vi "HW_Timings_Calibration.vi"(3 "Error In":errorcluster, 4 "Calibration SW timings":dbl[](array[numeric]), 5 "Calibration HW timings":u32[](array[numeric]), 6 "Settings cluster in":T1={"Defaults"={"Default User"=0.0, "VISA Resource Name "="Tracker"}, "Recording and saving"={"Researcher name"="Researcher", "Name prefix"="Track", "Data post-processing"={"Filter type"=enum."Savitzky-Golay", "Length"=31, "Order"=3}, "Stop at"=0.0, "\"Stop at\" enabled"=FALSE, "Default save folder path"=path "", "Acquisition FPS"=enum."Optimal"}, "Geometry"={"Cage diameter, mm"=180, "Starting angle MIDFIELD"=0, "Starting angle BORDER"=0, "Radius, mm CENTER"=30, "Radius, mm MIDFIELD"=75, "N segments MIDFIELD"=2, "N segments BORDER"=4, "R-gap, mm"=0.0, "Bridge swap"=FALSE, "Bridge H. offset"=0.0, "Bridge V. offset"=0.0, "Twisted neck"=FALSE, "Alt. magn. orientation"=FALSE}, "IO parameters"={"IO general config."=12, "IO 1 configuration"=1, "IO 2 configuration"=1, "IO 3 configuration"=0, "IO 4 configuration"=0, "Activate ext. RS-232"=0, "IO inversion config."=0, "Sync capability"=1}, "Stimulus presets array"=[{"Event type"=0, "Dur., s"=0.0, "Stim., s"=0.0, "TTL out N"=1, "Set/Clear"=FALSE, "Stim. has been set"=FALSE}, {"Event type"=0, "Dur., s"=0.0, "Stim., s"=0.0, "TTL out N"=1, "Set/Clear"=FALSE, "Stim. has been set"=FALSE}, {"Event type"=0, "Dur., s"=0.0, "Stim., s"=0.0, "TTL out N"=1, "Set/Clear"=FALSE, "Stim. has been set"=FALSE}, {"Event type"=0, "Dur., s"=0.0, "Stim., s"=0.0, "TTL out N"=1, "Set/Clear"=FALSE, "Stim. has been set"=FALSE}, {"Event type"=0, "Dur., s"=0.0, "Stim., s"=0.0, "TTL out N"=1, "Set/Clear"=FALSE, "Stim. has been set"=FALSE}, {"Event type"=0, "Dur., s"=0.0, "Stim., s"=0.0, "TTL out N"=1, "Set/Clear"=FALSE, "Stim. has been set"=FALSE}, {"Event type"=0, "Dur., s"=0.0, "Stim., s"=0.0, "TTL out N"=1, "Set/Clear"=FALSE, "Stim. has been set"=FALSE}, {"Event type"=0, "Dur., s"=0.0, "Stim., s"=0.0, "TTL out N"=1, "Set/Clear"=FALSE, "Stim. has been set"=FALSE}, {"Event type"=0, "Dur., s"=0.0, "Stim., s"=0.0, "TTL out N"=1, "Set/Clear"=FALSE, "Stim. has been set"=FALSE}, {"Event type"=0, "Dur., s"=0.0, "Stim., s"=0.0, "TTL out N"=1, "Set/Clear"=FALSE, "Stim. has been set"=FALSE}, {"Event type"=0, "Dur., s"=0.0, "Stim., s"=0.0, "TTL out N"=1, "Set/Clear"=FALSE, "Stim. has been set"=FALSE}, {"Event type"=0, "Dur., s"=0.0, "Stim., s"=0.0, "TTL out N"=1, "Set/Clear"=FALSE, "Stim. has been set"=FALSE}, {"Event type"=0, "Dur., s"=0.0, "Stim., s"=0.0, "TTL out N"=1, "Set/Clear"=FALSE, "Stim. has been set"=FALSE}, {"Event type"=0, "Dur., s"=0.0, "Stim., s"=0.0, "TTL out N"=1, "Set/Clear"=FALSE, "Stim. has been set"=FALSE}], "Calibration parameters"={"Timing calibration sw/hw"=1.0, "True FPS"=80.0, "Disp. calibration info"=[]}, "Settings loaded OK"=FALSE} {"Calibration parameters"."Disp. calibration info"."Speed, µl per ms" format="%.3g"; "Calibration parameters"."True FPS" format="%.10g"; "Calibration parameters"."Timing calibration sw/hw" format="%.10g"; "Stimulus presets array"."Event type" items=["Stay for N seconds"]; "Stimulus presets array"."TTL out N" items=["1"=1, "2"=2, "1+2"=3]; "Recording and saving"."Data post-processing"."Order" min=3 max=11 step=2; "Recording and saving"."Data post-processing"."Length" min=5 max=301 step=2; "Geometry"."Cage diameter, mm" scale=0.0..340.0}) -> (0 "Error out":T9, 1 "Calibration information":string, 2 "Settings cluster out":T1={"Defaults"={"Default User"=0.0, "VISA Resource Name "="Tracker"}, "Recording and saving"={"Researcher name"="Researcher", "Name prefix"="Track", "Data post-processing"={"Filter type"=enum."Savitzky-Golay", "Length"=31, "Order"=3}, "Stop at"=0.0, "\"Stop at\" enabled"=FALSE, "Default save folder path"=path "", "Acquisition FPS"=enum."Optimal"}, "Geometry"={"Cage diameter, mm"=180, "Starting angle MIDFIELD"=0, "Starting angle BORDER"=0, "Radius, mm CENTER"=30, "Radius, mm MIDFIELD"=75, "N segments MIDFIELD"=2, "N segments BORDER"=4, "R-gap, mm"=0.0, "Bridge swap"=FALSE, "Bridge H. offset"=0.0, "Bridge V. offset"=0.0, "Twisted neck"=FALSE, "Alt. magn. orientation"=FALSE}, "IO parameters"={"IO general config."=12, "IO 1 configuration"=1, "IO 2 configuration"=1, "IO 3 configuration"=0, "IO 4 configuration"=0, "Activate ext. RS-232"=0, "IO inversion config."=0, "Sync capability"=1}, "Stimulus presets array"=[{"Event type"=0, "Dur., s"=0.0, "Stim., s"=0.0, "TTL out N"=1, "Set/Clear"=FALSE, "Stim. has been set"=FALSE}, {"Event type"=0, "Dur., s"=0.0, "Stim., s"=0.0, "TTL out N"=1, "Set/Clear"=FALSE, "Stim. has been set"=FALSE}, {"Event type"=0, "Dur., s"=0.0, "Stim., s"=0.0, "TTL out N"=1, "Set/Clear"=FALSE, "Stim. has been set"=FALSE}, {"Event type"=0, "Dur., s"=0.0, "Stim., s"=0.0, "TTL out N"=1, "Set/Clear"=FALSE, "Stim. has been set"=FALSE}, {"Event type"=0, "Dur., s"=0.0, "Stim., s"=0.0, "TTL out N"=1, "Set/Clear"=FALSE, "Stim. has been set"=FALSE}, {"Event type"=0, "Dur., s"=0.0, "Stim., s"=0.0, "TTL out N"=1, "Set/Clear"=FALSE, "Stim. has been set"=FALSE}, {"Event type"=0, "Dur., s"=0.0, "Stim., s"=0.0, "TTL out N"=1, "Set/Clear"=FALSE, "Stim. has been set"=FALSE}, {"Event type"=0, "Dur., s"=0.0, "Stim., s"=0.0, "TTL out N"=1, "Set/Clear"=FALSE, "Stim. has been set"=FALSE}, {"Event type"=0, "Dur., s"=0.0, "Stim., s"=0.0, "TTL out N"=1, "Set/Clear"=FALSE, "Stim. has been set"=FALSE}, {"Event type"=0, "Dur., s"=0.0, "Stim., s"=0.0, "TTL out N"=1, "Set/Clear"=FALSE, "Stim. has been set"=FALSE}, {"Event type"=0, "Dur., s"=0.0, "Stim., s"=0.0, "TTL out N"=1, "Set/Clear"=FALSE, "Stim. has been set"=FALSE}, {"Event type"=0, "Dur., s"=0.0, "Stim., s"=0.0, "TTL out N"=1, "Set/Clear"=FALSE, "Stim. has been set"=FALSE}, {"Event type"=0, "Dur., s"=0.0, "Stim., s"=0.0, "TTL out N"=1, "Set/Clear"=FALSE, "Stim. has been set"=FALSE}, {"Event type"=0, "Dur., s"=0.0, "Stim., s"=0.0, "TTL out N"=1, "Set/Clear"=FALSE, "Stim. has been set"=FALSE}], "Calibration parameters"={"Timing calibration sw/hw"=1.0, "True FPS"=80.0, "Disp. calibration info"=[]}, "Settings loaded OK"=FALSE} {"Calibration parameters"."Disp. calibration info"."Speed, µl per ms" format="%.3g"; "Calibration parameters"."True FPS" format="%.10g"; "Calibration parameters"."Timing calibration sw/hw" format="%.10g"; "Stimulus presets array"."Event type" items=["Stay for N seconds"]; "Stimulus presets array"."TTL out N" items=["1"=1, "2"=2, "1+2"=3]; "Recording and saving"."Data post-processing"."Order" min=3 max=11 step=2; "Recording and saving"."Data post-processing"."Length" min=5 max=301 step=2; "Geometry"."Cage diameter, mm" scale=0.0..340.0})   [LabVIEW 2018, in "Tracker.lvlib"]
uses:
  Tracker.lvlib
  Controls/CTL_Settings_cluster.ctl
  Controls/CTL_Filter_selector.ctl
  Controls/CTL_Acquisition_speed_selector.ctl
  Controls/CTL_Segmented_plot_parameters.ctl
  Controls/CTL_IO_params_cluster.ctl
  Controls/CTL_Single_stimulus_setting.ctl
  Controls/CTL_Calibration_parameters.ctl
  Controls/CTL_Dispenser_calibration_info.ctl
  <vilib>/Utility/miscctls.llb/LVPointTypeDef.ctl
  <vilib>/Analysis/NI_AALBase.lvlib
panel:
  out "SW seconds in HW second":dbl format="%#.10g"
  in  "OK Button":bool
  out "True FPS":dbl format="%.3f"
  out "Avg. software frame time SD, ms":dbl format="%.3f"
  out "Avg. hardware frame time SD, ms":dbl format="%.3f"
  out "Avg. software frame time, ms":dbl format="%.3f"
  out "Avg. hardware frame time, ms":dbl format="%.3f"
  out "Frame delta time, ms":dbl[][](graph) caption="Waveform Chart - Light"
  # "Calibration information"
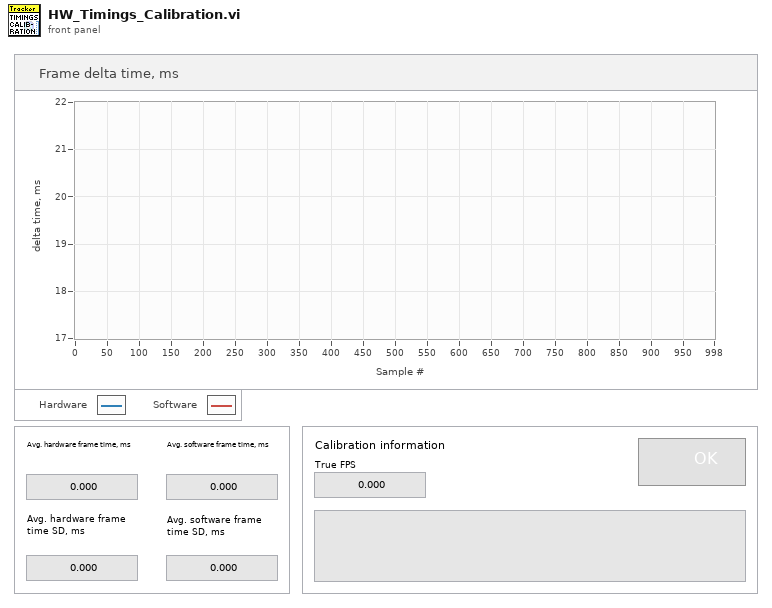
[diagram p1: front panel]
types:
  T1 = typedef "Tracker.lvlib/CTL_Settings_cluster.ctl" = cluster{"Defaults":cluster{"Default User":dbl, "VISA Resource Name ":string}, "Recording and saving":cluster{"Researcher name":string, "Name prefix":string, "Data post-processing":T2, "Stop at":dbl, "\"Stop at\" enabled":bool, "Default save folder path":path, "Acquisition FPS":T3}, "Geometry":T4, "IO parameters":T5, "Stimulus presets array":T6[], "Calibration parameters":T7, "Settings loaded OK":bool}
  T2 = typedef "Tracker.lvlib/CTL_Filter_selector.ctl" = cluster{"Filter type":enum16{"None", "Savitzky-Golay"}, "Length":i32, "Order":i32}
  T3 = typedef "Tracker.lvlib/CTL_Acquisition_speed_selector.ctl" = enum16{"Max", "Optimal", "Eco"}
  T4 = typedef "Tracker.lvlib/CTL_Segmented_plot_parameters.ctl" = cluster{"Cage diameter, mm":u16, "Starting angle MIDFIELD":i16, "Starting angle BORDER":i16, "Radius, mm CENTER":u16, "Radius, mm MIDFIELD":u16, "N segments MIDFIELD":u8, "N segments BORDER":u8, "R-gap, mm":sgl, "Bridge swap":bool, "Bridge H. offset":sgl, "Bridge V. offset":sgl, "Twisted neck":bool, "Alt. magn. orientation":bool}
  T5 = typedef "Tracker.lvlib/CTL_IO_params_cluster.ctl" = cluster{"IO general config.":u16, "IO 1 configuration":u16, "IO 2 configuration":u16, "IO 3 configuration":u16, "IO 4 configuration":u16, "Activate ext. RS-232":u16, "IO inversion config.":u16, "Sync capability":u8}
  T6 = typedef "Tracker.lvlib/CTL_Single_stimulus_setting.ctl" = cluster{"Event type":u16, "Dur., s":sgl, "Stim., s":sgl, "TTL out N":u16, "Set/Clear":bool, "Stim. has been set":bool}
  T7 = typedef "Tracker.lvlib/CTL_Calibration_parameters.ctl" = cluster{"Timing calibration sw/hw":dbl, "True FPS":dbl, "Disp. calibration info":T8}
  T8 = typedef "Tracker.lvlib/CTL_Dispenser_calibration_info.ctl" = cluster{"Channel":u8, "Speed, µl per ms":dbl}[]
  T9 = cluster{"Boolean Round":bool, "code":i32, "source":string}
  T10 = typedef "LVPointTypeDef.ctl" = cluster{"Horizontal":i16, "Vertical":i16}
  T11 = enum32{"invalid app kind", "Development System", "Run Time System", "Student Edition", "Embedded LabVIEW", "Evaluation", "Custom"}
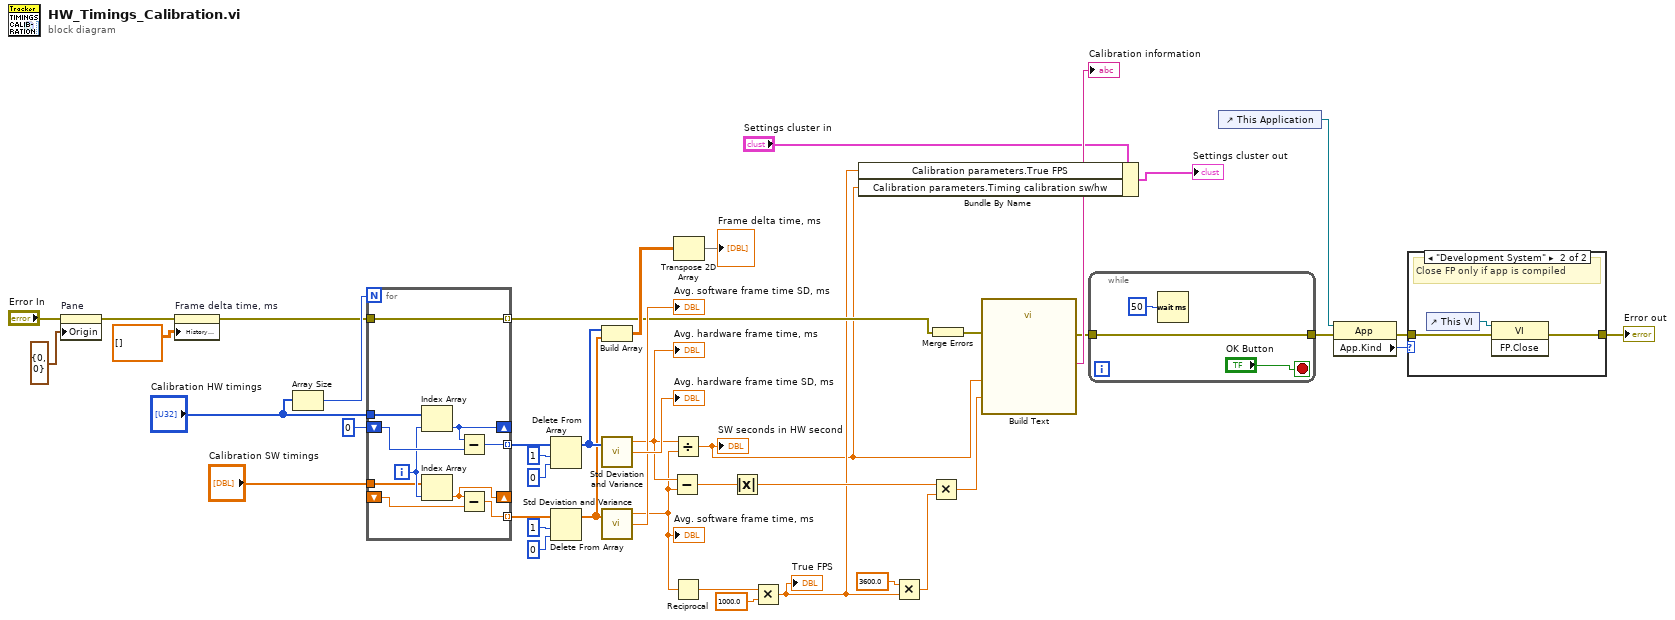
[diagram p0: block diagram]
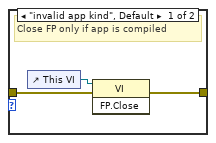
[diagram p2: hidden frame]
diagram:
  n1 = property on="Pane" class="Pane"(error in="Error In", "Origin"=T10 {"Horizontal"=0, "Vertical"=0}) -> (error out=w24:errorcluster)  [unwired: 1 in, 1 out]
  n2 = property on="Frame delta time, ms" class="WFChart (strict)"(error in=w24, "History Data"=dbl[][] []) -> (error out=w23:errorcluster)  [unwired: 1 in, 1 out]
  n3 = Array Size(array="Calibration HW timings") -> (size(s)=w41:i32)
  n4 = for {
    N: w41 -> [_]
    tunnel: "Calibration HW timings" -> [w53]
    tunnel: "Calibration SW timings" -> [w48]
    shift-right: [w52] -> _
    shift-left: u32 0 ("value out") -> [w51]
    tunnel: [w50] -> w39 mode=indexing
    shift-right: [w46] -> _
    shift-left: _ -> [w47]
    tunnel: [w45] -> w34 mode=indexing
    tunnel: w23 -> [w44]
    tunnel: [w44] -> w21 mode=indexing
    i -> [w49]
    n5 = Index Array(array=w53, index=w49) -> (element=w52:u32)
    n6 = Index Array(array=w48, index=w49) -> (element=w46:dbl)
    n7 = Subtract(x=w52, y=w51) -> (x-y=w50:u32)
    n8 = Subtract(x=w46, y=w47) -> (x-y=w45:dbl)
  }
  n9 = Delete From Array(array=w39, length=1, index=0) -> (array with subset deleted=w30:u32[])  [unwired: 1 out]
  n10 = Delete From Array(array=w34, length=1, index=0) -> (array with subset deleted=w29:dbl[])  [unwired: 1 out]
  n11 = Build Array(w30, w29) -> (w33:dbl[][])
  n12 = call <vilib>:"Std Deviation and Variance.vi"("X"=w30) -> ("mean"=w11:dbl, "standard deviation"=→"Avg. hardware frame time SD, ms":dbl)  [unwired: 1 in, 1 out]
  "Avg. hardware frame time, ms" <- w11
  n13 = call <vilib>:"Std Deviation and Variance.vi"("X"=w29) -> ("mean"=w5:dbl, "standard deviation"=→"Avg. software frame time SD, ms":dbl)  [unwired: 1 in, 1 out]
  "Avg. software frame time, ms" <- w5
  n14 = Subtract(x=w11, y=w5) -> (x-y=w10:dbl)
  n15 = Divide(x=w11, y=w5) -> (x/y=w2:dbl)
  "SW seconds in HW second" <- w2
  n16 = Reciprocal(x=w5) -> (1/x=w26:dbl)
  n17 = Transpose 2D Array(2D array=w33) -> (transposed array=→"Frame delta time, ms":dbl[][])
  n18 = Absolute Value(x=w10) -> (abs(x)=w9:dbl)
  n19 = Multiply(x=w26, y=1000.0) -> (x*y=w3:dbl)
  "True FPS" <- w3
  n20 = Bundle By Name(cluster="Settings cluster in", "Calibration parameters.True FPS"=w3, "Calibration parameters.Timing calibration sw/hw"=w2) -> (→"Settings cluster out":T1)
  n21 = Multiply(x=3600.0, y=w3) -> (x*y=w6:dbl)
  n22 = Multiply(x=w9, y=w6) -> (x*y=w8:dbl)
  n23 = Merge Errors(w21) -> (w20:errorcluster)
  n24 = call "Build Text"("swsec"=w2, "msec"=w8, "error in (no error)"=w20) -> ("Result"=→"Calibration information":string, "error out"=w17:errorcluster)  [unwired: 11 in]
  n25 = while {
    tunnel: [w54] -> w15
    tunnel: w17 -> [w54]
    stop <- "OK Button" stop-if-true
    n26 = Wait (ms)(milliseconds to wait=u32 50) -> ()  [unwired: 1 out]
  }
  n27 = control-ref of="This Application"() -> (w12:refnum<vi>)
  n28 = property class="App"(reference=w12, error in=w15) -> (error out=w14:errorcluster, "App.Kind"=w16:T11)  [unwired: 1 out]
  n29 = case shown="\"Development System\"" w16 {
    tunnel: w14 -> [w59 w62]
    tunnel: [w58 w61] -> w13
    frame "invalid app kind", Default {
      # "Close FP only if app is compiled"
      n30 = control-ref of="This VI"() -> (w57:refnum<vi>)
      n31 = invoke class="VI" method="FP.Close"(reference=w57, error in=w59) -> (error out=w58:errorcluster)  [unwired: 1 in, 2 out]
    }
    frame "Development System" {
      # "Close FP only if app is compiled"
      n32 = control-ref of="This VI"() -> (w60:refnum<vi>)
      n33 = invoke class="VI" method="FP.Close"(reference=w60, error in=w62) -> (error out=w61:errorcluster)  [unwired: 1 in, 2 out]
    }
  }
  "Error out" <- w13
